vi "Browse for XNET Database.vi"(8 "error in (no error)":errorcluster) -> (0 "error out":errorcluster, 2 "Cancel Out":bool, 3 "XNET Settings":T1={"Database"="", "Cluster"="", "Port"="", "Baud rate [Bd]"=0, "Termination"=0, "CAN I/O Mode"=0, "FD Baud rate [Bd]"=500000, "Priority"=100, "Use Legacy"=FALSE} {"CAN I/O Mode" items=["CAN 2.0", "CAN FD", "CAN FD+BRS"]; "Termination" items=["Off", "On"]})   [LabVIEW 2019, in "Protection and Counter Addon System Explorer.lvlib"]
uses:
  Protection and Counter Addon System Explorer.lvlib
  Shared/Types/XNET Settings.ctl
  <resource>/objmgr/xnet.rc
  Shared/Protection and Counter Addon Shared.lvlib
panel:
  in  "FD Baud rate [Bd]":u64=500000
  in  "CAN I/O Mode":u32(ring) items=["CAN 2.0", "CAN FD", "CAN FD+BRS"]
  in  "Baud rate [Bd]":u64=500000
  in  "Select CAN Cluster":u16(ring)
  in  "Cancel":bool
  in  "Select":bool
  in  "XNET Database":refnum<k21>
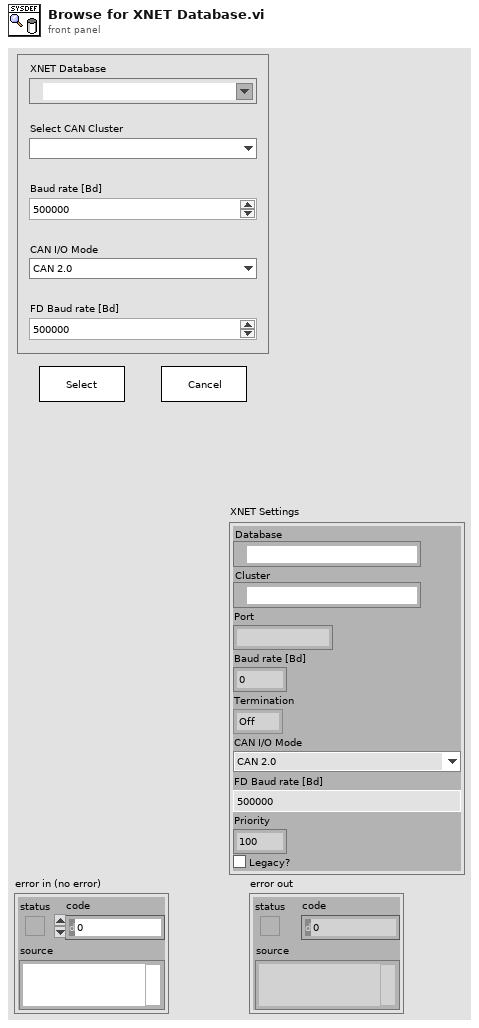
[diagram p1: front panel]
types:
  T1 = typedef "Protection and Counter Addon Shared.lvlib/XNET Settings.ctl" = cluster{"Database":refnum<k21>, "Cluster":refnum<k21>, "Port":string, "Baud rate [Bd]":u64, "Termination":u32, "CAN I/O Mode":u32, "FD Baud rate [Bd]":u64, "Priority":i32, "Use Legacy":bool}
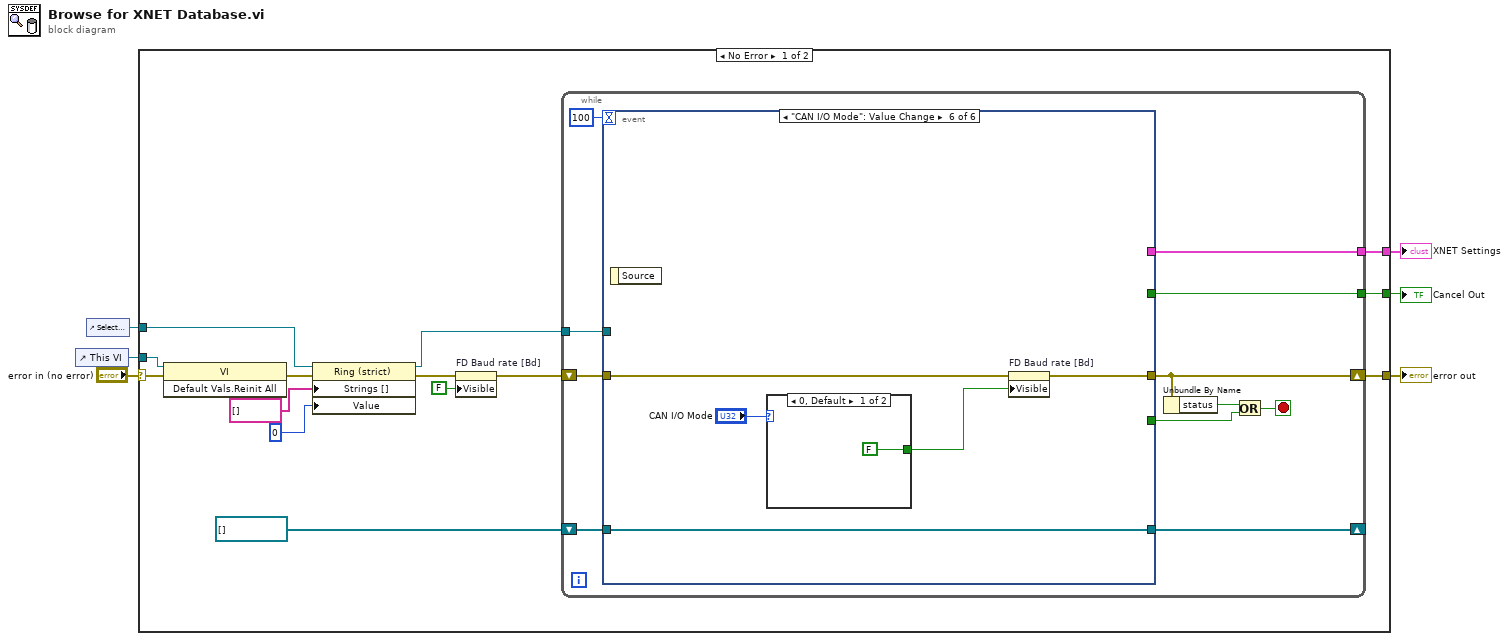
[diagram p0: block diagram]
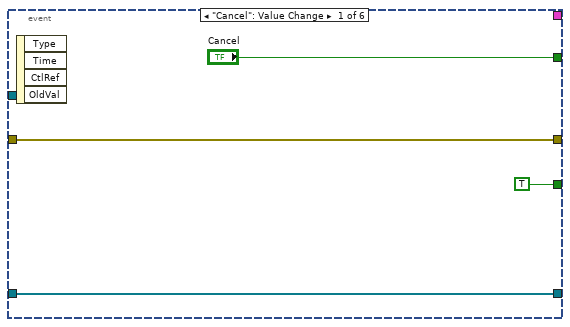
[diagram p2: hidden frame]
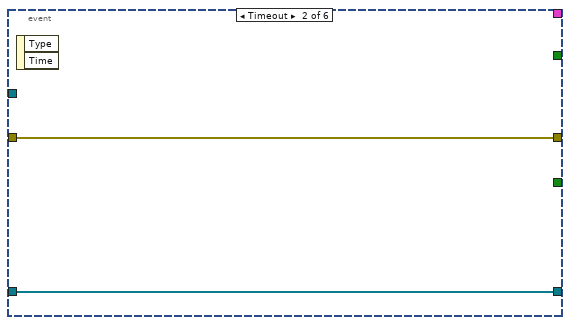
[diagram p3: hidden frame]
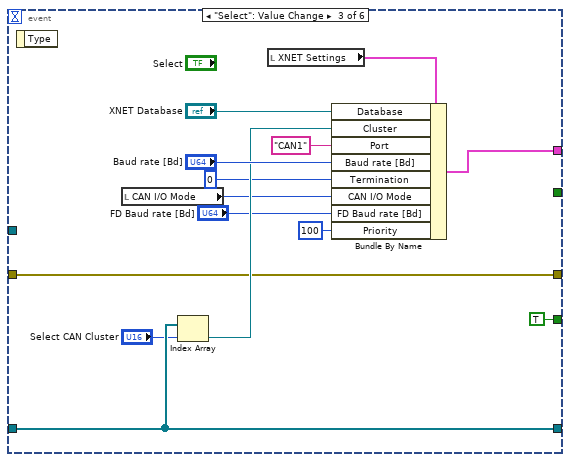
[diagram p4: hidden frame]
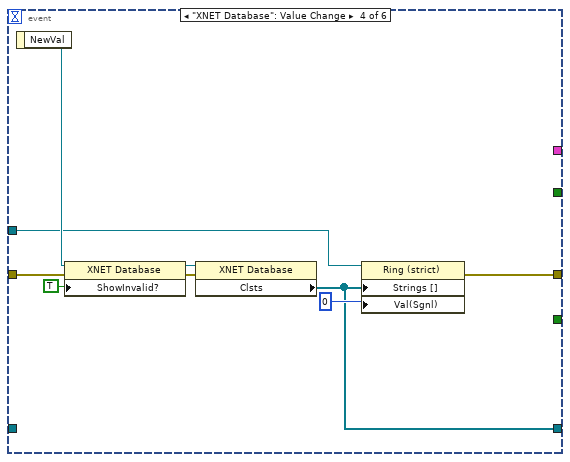
[diagram p5: hidden frame]
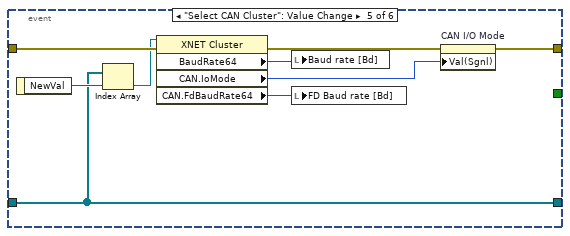
[diagram p6: hidden frame]
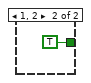
[diagram p7: hidden frame]
diagram:
  n1 = control-ref of="This VI"() -> (w3:refnum<vi>)
  n2 = control-ref of="Select CAN Cluster"() -> (w1:refnum<vi>)
  n3 = case shown="No Error" "error in (no error)" {
    selector: "error in (no error)" -> [w19 w77]
    tunnel: [w17 w77] -> w5
    tunnel: [w20 _] -> w4
    tunnel: w3 -> [w18 _]
    tunnel: [w15 _] -> w2
    tunnel: w1 -> [w14 _]
    frame No Error {
      n4 = invoke class="VI" method="Default Vals.Reinit All"(reference=w18, error in=w19) -> (error out=w13:errorcluster)  [unwired: 1 in, 2 out]
      n5 = property on="Property Node" class="Ring (strict)"(reference=w14, error in=w13, "Strings []"=string[] [], "Value"=u16 0) -> (reference out=w12:refnum<vi>, error out=w9:errorcluster)
      n6 = property on="FD Baud rate [Bd]" class="DigNum (strict)"(error in=w9, "Visible"=FALSE) -> (error out=w8:errorcluster)  [unwired: 1 in, 1 out]
      n7 = while {
        tunnel: [w31] -> w20
        shift-right: [w29] -> _
        shift-left: refnum<k21>[] [] ("Clsts") -> [w28]
        shift-right: [w25] -> w17
        shift-left: w8 -> [w30]
        tunnel: [w27] -> w15
        tunnel: w12 -> [w21]
        stop <- w22 stop-if-true
        n8 = event shown="[5] \"CAN I/O Mode\": Value Change" {
          selector: _ -> [_ _ _ _ _ _]
          dyn-events: _ -> [_ _ _ _ _ _]
          timeout: 100 -> [_ _ _ _ _ _]
          tunnel: ["Cancel" _ _ _ _ _] -> w31
          tunnel: w30 -> [w33 w37 w43 w57 w68 w74]
          tunnel: [w34 w36 w48 w54 w65 w72] -> w29
          tunnel: w28 -> [w34 w36 w48 _ w65 w72]
          tunnel: [w33 w37 w43 w52 w63 w73] -> w25
          tunnel: [_ _ w45 _ _ _] -> w27
          tunnel: [TRUE _ TRUE _ _ _] -> w23
          tunnel: w21 -> [_ _ _ w53 _ _]
          event "Cancel": Value Change {
            n9 = event-data() -> ()  [unwired: 1 in, 4 out]
          }
          event Timeout {
            n10 = event-data() -> ()  [unwired: 1 in, 2 out]
          }
          event "Select": Value Change {
            n11 = event-data() -> ()  [unwired: 1 in, 1 out]
            n12 = local read "CAN I/O Mode"() -> (w38:u32)
            n13 = Index Array(array=w48, index="Select CAN Cluster") -> (element=w46:refnum<k21>)
            n14 = local read "XNET Settings"() -> (w49:T1)
            n15 = Bundle By Name(cluster=w49, "Database"="XNET Database", "Cluster"=w46, "Port"="CAN1", "Baud rate [Bd]"="Baud rate [Bd]", "Termination"=u32 0, "CAN I/O Mode"=w38, "FD Baud rate [Bd]"="FD Baud rate [Bd]", "Priority"=100) -> (w45:T1)
          }
          event "XNET Database": Value Change {
            n16 = event-data() -> ("NewVal"=w56:refnum<k21>)  [unwired: 1 in]
            n17 = property class="XNET Database"(reference=w56, error in=w57, "ShowInvalid?"=TRUE ("Show Invalid From Open?")) -> (reference out=w60:refnum<k21>, error out=w59:errorcluster)
            n18 = property class="XNET Database"(reference=w60, error in=w59) -> ("Clsts"=w54:refnum<k21>[])  [unwired: 2 out]
            n19 = property on="Property Node" class="Ring (strict)"(reference=w53, "Strings []"=w54, "Val(Sgnl)"=u16 0 ("Value (Signaling)")) -> (error out=w52:errorcluster)  [unwired: 1 in, 1 out]
          }
          event "Select CAN Cluster": Value Change {
            n20 = event-data() -> ("NewVal"=w67:u16)  [unwired: 1 in]
            n21 = Index Array(array=w65, index=w67) -> (element=w66:refnum<k21>)
            n22 = property class="XNET Cluster"(reference=w66, error in=w68) -> (error out=w62:errorcluster, "BaudRate64"=w69:u64, "CAN.IoMode"=w61:u32, "CAN.FdBaudRate64"=w64:u64)  [unwired: 1 out]
            n23 = local write "Baud rate [Bd]"(w69) -> ()
            n24 = local write "FD Baud rate [Bd]"(w64) -> ()
            n25 = property on="CAN I/O Mode" class="Ring (strict)"(error in=w62, "Val(Sgnl)"=w61) -> (error out=w63:errorcluster)  [unwired: 1 in, 1 out]
          }
          event "CAN I/O Mode": Value Change {
            n26 = event-data() -> ()  [unwired: 1 in, 1 out]
            n27 = case shown="0, Default" "CAN I/O Mode" {
              tunnel: [FALSE TRUE] -> w70
              frame 0, Default {
              }
              frame 1, 2 {
              }
            }
            n28 = property on="FD Baud rate [Bd]" class="DigNum (strict)"(error in=w74, "Visible"=w70) -> (error out=w73:errorcluster)  [unwired: 1 in, 1 out]
          }
        }
        n29 = Unbundle By Name(w25) -> ("status"=w24:bool)
        n30 = Or(x=w24, y=w23) -> (x .or. y?=w22:bool)
      }
    }
    frame Error {
    }
  }
  "error out" <- w5
  "Cancel Out" <- w4
  "XNET Settings" <- w2
